vi "Data.Engine.ReInitialize.vi"(8 "error in":errorcluster, 11 "Compiled.InlineAsync.Settings":T3 {"Read"."Refs"."Data Reference" format="%.0x"; "Write"."Refs"."Data Reference" format="%.0x"; "ReadWrite"."Refs" format="%.0x"}) -> (0 "error out":errorcluster, 3 "Data Access Engine":refnum<class "Data Access Engine.lvclass">)   [LabVIEW 2023, in "Data Access Engine.lvlib" / "Data Access Engine.lvclass"]
uses:
  Data Access Engine.lvclass
  Access Type Classes/Read/Read.lvclass
  Access Type Classes/Write/Write.lvclass
  Access Type Classes/ReadWrite/ReadWrite.lvclass
  Data Access Engine.lvclass/Data Access Engine.ctl
  <vilib>/NI VeriStand/Custom Device API/Data Reference.ctl
  <vilib>/NI VeriStand/Custom Device API/Custom Device API.lvlib
  <vilib>/NI VeriStand/Custom Device API/Block Data Reference.ctl
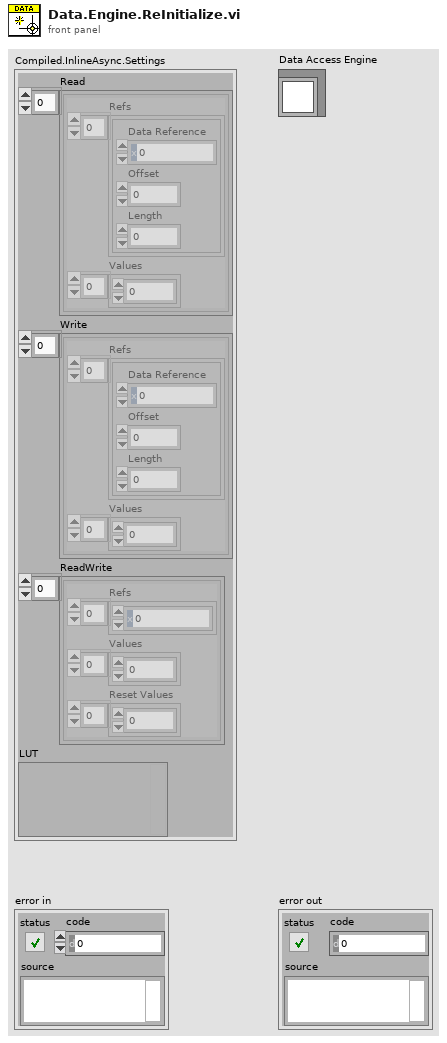
[diagram p1: front panel]
types:
  T1 = typedef "Custom Device API.lvlib/Block Data Reference.ctl" = cluster{"Data Reference":T2, "Offset":u64, "Length":u64}
  T2 = typedef "Custom Device API.lvlib/Data Reference.ctl" = i32
  T3 = cluster{"Read":cluster{"Refs":T1[], "Values":dbl[]}[], "Write":cluster{"Refs":T1[], "Values":dbl[]}[], "ReadWrite":cluster{"Refs":T2[], "Values":dbl[], "Reset Values":dbl[]}[], "LUT":variant}
  T4 = cluster{"Refs":T2[], "Values":dbl[], "Reset Values":dbl[]}[]
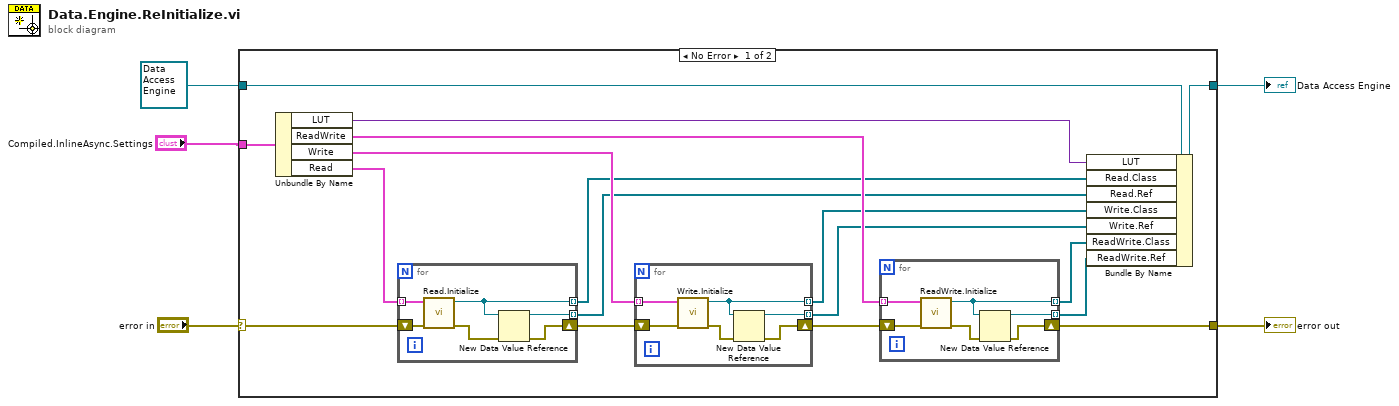
[diagram p0: block diagram]
diagram:
  n1 = case shown="No Error" "error in" {
    selector: "error in" -> [w22 w42]
    tunnel: [w19 w42] -> w4
    tunnel: [w12 w41] -> w3
    tunnel: refnum<class "Data Access Engine.lvclass"> refnum ("Data Access API.lvlib:Data Access API.lvclass") -> [w7 w41]
    tunnel: "Compiled.InlineAsync.Settings" -> [w8 _]
    frame No Error {
      n2 = Unbundle By Name(w8) -> ("LUT"=w6:variant, "ReadWrite"=w16:T4, "Write"=w17:cluster{"Refs":T1[], "Values":dbl[]}[], "Read"=w18:cluster{"Refs":T1[], "Values":dbl[]}[])
      n3 = for {
        tunnel: w18 -> [w37] mode=indexing
        shift-right: [w38] -> w21
        shift-left: w22 -> [w40]
        tunnel: [w36] -> w13 mode=indexing
        tunnel: [w35] -> w9 mode=indexing
        n4 = call "Read.Initialize.vi"("error in (no error)"=w40, "Settings"=w37) -> ("error out"=w39:errorcluster, "Read out"=w36:refnum<class "Read.lvclass">)  [unwired: 8 in]
        n5 = New Data Value Reference(data value=w36, error in=w39) -> (data value reference=w35:refnum<data-value>, error out=w38:errorcluster)
      }
      n6 = for {
        tunnel: w17 -> [w31] mode=indexing
        shift-right: [w32] -> w20
        shift-left: w21 -> [w34]
        tunnel: [w30] -> w14 mode=indexing
        tunnel: [w29] -> w10 mode=indexing
        n7 = call "Write.Initialize.vi"("error in (no error)"=w34, "Settings"=w31) -> ("error out"=w33:errorcluster, "Write out"=w30:refnum<class "Write.lvclass">)  [unwired: 8 in]
        n8 = New Data Value Reference(data value=w30, error in=w33) -> (data value reference=w29:refnum<data-value>, error out=w32:errorcluster)
      }
      n9 = for {
        tunnel: w16 -> [w25] mode=indexing
        shift-right: [w26] -> w19
        shift-left: w20 -> [w28]
        tunnel: [w24] -> w15 mode=indexing
        tunnel: [w23] -> w11 mode=indexing
        n10 = call "ReadWrite.Initialize.vi"("error in (no error)"=w28, "Settings"=w25) -> ("error out"=w27:errorcluster, "ReadWrite out"=w24:refnum<class "ReadWrite.lvclass">)  [unwired: 8 in]
        n11 = New Data Value Reference(data value=w24, error in=w27) -> (data value reference=w23:refnum<data-value>, error out=w26:errorcluster)
      }
      n12 = Bundle By Name(cluster=w7, "LUT"=w6, "Read.Class"=w13, "Read.Ref"=w9, "Write.Class"=w14, "Write.Ref"=w10, "ReadWrite.Class"=w15, "ReadWrite.Ref"=w11) -> (w12:refnum<class "Data Access Engine.lvclass">)
    }
    frame Error {
    }
  }
  "error out" <- w4
  "Data Access Engine" <- w3
